vi "GBL_variables.vi"() -> ()   [LabVIEW 2017]
panel:
  in  "Y_end":dbl
  in  "X_end":dbl
  in  "Map_Forget_factor":dbl
  in  "Const_V":dbl
  in  "Const_V_range(m)":dbl=0.3
  in  "Obs_avoid_length_angle_index":dbl
  in  "Obs_avoid_start_angle_index":dbl
  in  "log_odd_sensor_detected":dbl
  in  "K_theta":dbl
  in  "K_d":dbl
  in  "Init_Distance_goal":dbl
  in  "Y_goal":dbl
  in  "X_goal":dbl
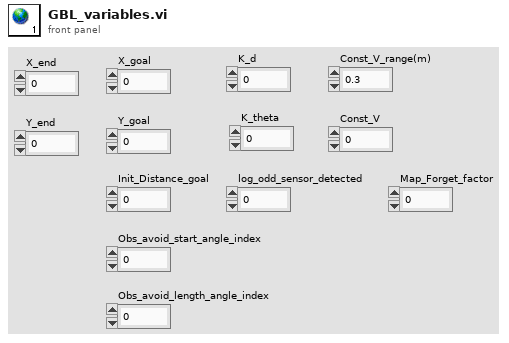
[diagram p1: front panel]
diagram:
